vi "S2C_PCIe1762H_Proc_DigitalReadAll.vi"(8 "Error In":errorcluster) -> (0 "Error Out":errorcluster)   [LabVIEW 2024]
uses:
  S2C_PCIe1762H_Proc_Globals.vi
  <userlib>/DAQNavi Polymorphic VI/create/DAQNavi Create Channel(DO-Digital Output).vi
  <userlib>/DAQNavi Polymorphic VI/read/DAQNavi Read (Digital 1D U8 NChan 1Samp).vi
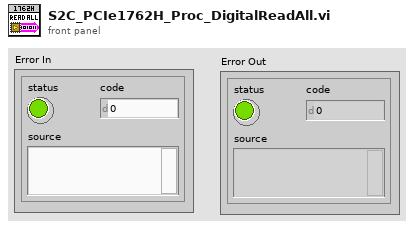
[diagram p1: front panel]
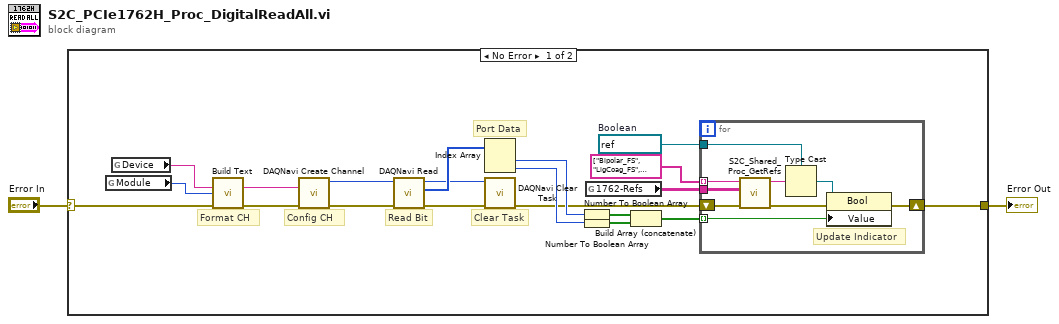
[diagram p0: block diagram]
diagram:
  n1 = case shown="No Error" "Error In" {
    selector: "Error In" -> [w4 w32]
    tunnel: [w3 w32] -> w1
    frame No Error {
      w16 = refnum<vi> refnum  # Boolean
      # "Port Data"
      # "Clear Task"
      # "Read Bit"
      # "Format CH"
      # "Config CH"
      n2 = global read "S2C_PCIe1762H_Proc_Globals.vi" "Module"() -> (w8:i32)
      n3 = global read "S2C_PCIe1762H_Proc_Globals.vi" "Device"() -> (w9:string)
      n4 = call "Build Text"("Device"=w9, "Module"=w8, "error in (no error)"=w4) -> ("Result"=w6:string, "error out"=w5:errorcluster)  [unwired: 11 in]
      n5 = call-poly <userlib>:"DAQNavi Create Channel.vi"("physical channels"=w6, "error in (no error)"=w5) -> ("task out"=w11:i32, "error out"=w10:errorcluster)  [unwired: 3 in, 9 out]
      n6 = call-poly <userlib>:"DAQNavi Read.vi"("error in (no error)"=w10, "task in"=w11) -> ("error out"=w12:errorcluster, "data"=w17:u8[], "task out"=w7:i32)  [unwired: 1 in, 6 out]
      n7 = Index Array(array=w17) -> (element #1=w18:u8, element #2=w19:u8)  [unwired: 2 in]
      n8 = call <userlib>:"DAQNavi Clear Task.vi"("error in (no error)"=w12, "task in"=w7) -> ("error out"=w13:errorcluster)  [unwired: 1 out]
      n9 = Number To Boolean Array(number=w18) -> (Boolean array=w20:bool[])
      n10 = Number To Boolean Array(number=w19) -> (Boolean array=w21:bool[])
      n11 = global read "S2C_PCIe1762H_Proc_Globals.vi" "1762-Refs"() -> (w15:string[][])
      n12 = Build Array (concatenate)(w20, w21) -> (w22:bool[])
      n13 = for {
        tunnel: string[] ["Bipolar_FS", "LigCoag_FS", "LigBipolar_FS", "LigSeal_FS", "LigCut_FS", "LigSpare_FS", "Mono2Coag_FS", "Mono2Cut_FS", "Mono2VL_FS", "Mono2Spare_FS", "Mono1Coag_FS", "Mono1Cut_FS", "Spare1", "Spare2", "Spare3", "Spare4"] -> [w29] mode=indexing
        tunnel: w15 -> [w30]
        shift-right: [w28] -> w3
        shift-left: w13 -> [w31]
        tunnel: w16 -> [w27]
        tunnel: w22 -> [w23] mode=indexing
        # "Update Indicator"
        n14 = call "S2C_Shared_Proc_GetRefs.vi"("Error In"=w31, "Refs"=w30, "Label"=w29) -> ("Error Out"=w25:errorcluster, "Reference"=w24:string)  [unwired: 7 in]
        n15 = Type Cast(type=w27, x=w24) -> (*(type *) &x=w26:refnum<vi>)
        n16 = property class="Bool"(reference=w26, error in=w25, "Value"=w23) -> (error out=w28:errorcluster)  [unwired: 1 out]
      }
    }
    frame Error {
    }
  }
  "Error Out" <- w1
